vi "3.1Test.vi"(8 "error in (no error)":errorcluster) -> (0 "error out":errorcluster)   [LabVIEW 2017]
uses:
  <vilib>/addons/_JKI Toolkits/Caraya/classes/Assert/Assert Equal Value_Variant.vi
  <vilib>/addons/_JKI Toolkits/Caraya/classes/Test/Test.lvclass
  <vilib>/addons/_JKI Toolkits/Caraya/classes/Assert/Assert.lvclass
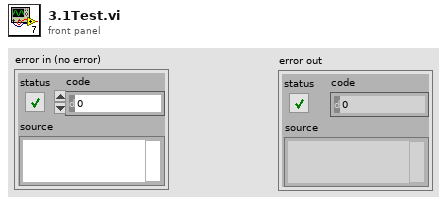
[diagram p1: front panel]
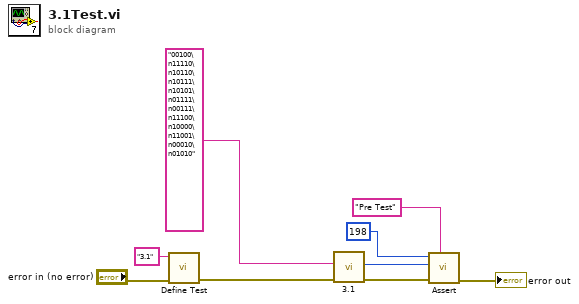
[diagram p0: block diagram]
diagram:
  n1 = call <vilib>:"Define Test.vi"("error in (no error)"="error in (no error)", "Label (VI Title)"="3.1") -> ("error out"=w7:errorcluster)  [unwired: 9 in]
  n2 = call "3.1.vi"("error in (no error)"=w7, "String"="00100\n11110\n10110\n10111\n10101\n01111\n00111\n11100\n10000\n11001\n00010\n01010") -> ("error out"=w6:errorcluster, "Numeric"=w5:i32)  [unwired: 8 in]
  n3 = call-poly <vilib>:"Assert.vi"("Label"="Pre Test", "error in (no error)"=w6, "Y"=w5, "X"=198 ("Numeric")) -> ("error out"=→"error out":errorcluster)  [unwired: 7 in]
